vi "Bootstrap Array with Linked Array.vi"(9 "Linked Array in":dbl[](array[numeric]), 11 "Array in":dbl[](array[numeric])) -> (1 "Linked Array out":dbl[](array[numeric]), 3 "Bootstrapped Array":dbl[](array[numeric]))   [LabVIEW 2021, in "Arrays.lvlib"]
uses:
  <vilib>/gmath/statdist.llb/Uniform (Discrete) Random.vi
  Arrays.lvlib
  <vilib>/gmath/NI_Gmath.lvlib
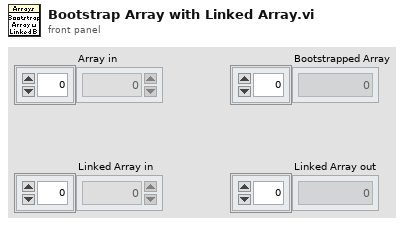
[diagram p1: front panel]
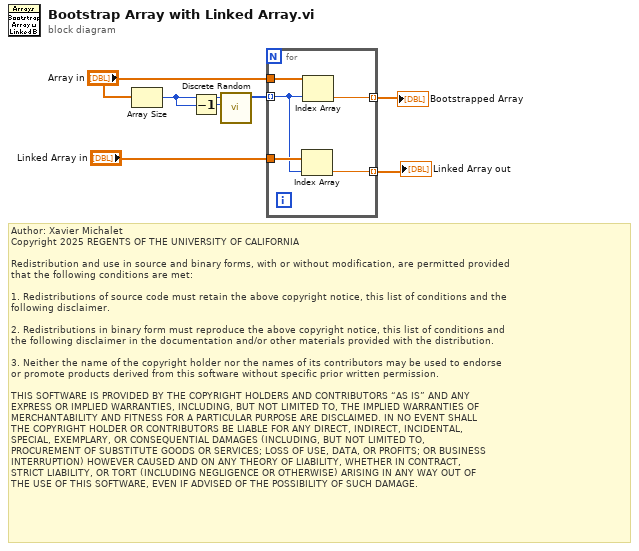
[diagram p0: block diagram]
diagram:
  # "Author: Xavier Michalet\nCopyright 2025 REGENTS OF THE UNIVERSITY OF CALIFORNIA\n\nRedistribution and use in source and binary forms, with or without modification, are permitted provided\nthat the following conditions are met:\n\n1. Redistributions of source code must retain the above copyright notice, this list of conditions and the\nfollowing disclaimer.\n\n2. Redistributions in binary form must reproduce the above copyright notice, this list of conditions and\nthe following disclaimer in the documentation and/or other materials provided with the distribution.\n\n3. Neither the name of the copyright holder nor the names of its contributors may be used to endorse \nor promote products derived from this software without specific prior written permission.\n\nTHIS SOFTWARE IS PROVIDED BY THE COPYRIGHT HOLDERS AND CONTRIBUTORS “AS IS” AND ANY \nEXPRESS OR IMPLIED WARRANTIES, INCLUDING, BUT NOT LIMITED TO, THE IMPLIED WARRANTIES OF\nMERCHANTABILITY AND FITNESS FOR A PARTICULAR PURPOSE ARE DISCLAIMED. IN NO EVENT SHALL\nTHE COPYRIGHT HOLDER OR CONTRIBUTORS BE LIABLE FOR ANY DIRECT, INDIRECT, INCIDENTAL, \nSPECIAL, EXEMPLARY, OR CONSEQUENTIAL DAMAGES (INCLUDING, BUT NOT LIMITED TO, \nPROCUREMENT OF SUBSTITUTE GOODS OR SERVICES; LOSS OF USE, DATA, OR PROFITS; OR BUSINESS\nINTERRUPTION) HOWEVER CAUSED AND ON ANY THEORY OF LIABILITY, WHETHER IN CONTRACT, \nSTRICT LIABILITY, OR TORT (INCLUDING NEGLIGENCE OR OTHERWISE) ARISING IN ANY WAY OUT OF\nTHE USE OF THIS SOFTWARE, EVEN IF ADVISED OF THE POSSIBILITY OF SUCH DAMAGE."
  n1 = Array Size(array="Array in") -> (size(s)=w7:i32)
  n2 = Decrement(x=w7) -> (x-1=w6:i32)
  n3 = call-poly <vilib>:"Discrete Random.vi"("n"=w6, "samples"=w7) -> ("uniform (discrete) random data"=w4:i32[])  [unwired: 8 in, 1 out]
  n4 = for {
    tunnel: "Array in" -> [w12]
    tunnel: w4 -> [w10] mode=indexing
    tunnel: "Linked Array in" -> [w11]
    tunnel: [w9] -> w2 mode=indexing
    tunnel: [w8] -> w1 mode=indexing
    n5 = Index Array(array=w11, index=w10) -> (element=w8:dbl)
    n6 = Index Array(array=w12, index=w10) -> (element=w9:dbl)
  }
  "Linked Array out" <- w1
  "Bootstrapped Array" <- w2
